vi "Agilent Scan EZ Temperature.vi"(0 "VISA Resource Name":refnum<visa-resource-name>, 2 "Control":enum16{"Initialize", "Read", "Experiment"}(ring), 5 "Channel Input":string, 11 "error in (no error)":errorcluster) -> (4 "VISA Resource Name Out":refnum<visa-resource-name>, 6 "read buffer":string, 8 "Output Array":dbl[](array[numeric]) format="%.2f", 15 "error out":errorcluster)   [LabVIEW 2012]
doc: "This VI lets you take simple temperature measurements. You can use various types of thermocouples, thermistors, or RTDs."
uses:
  Drivers/Agilent 34970/Agilent 34970.lvlib
panel:
  in  "Integration Time":u16(ring)=300 items=[".02 PLC"=10000, ".2 PLC"=1000, "1 PLC"=300, "2 PLC"=220, "10 PLC"=100, "20 PLC"=80, "100 PLC"=30, "200 PLC"=22]
  in  "AutoZero":bool
  out "Command":string
  out "Length":i32
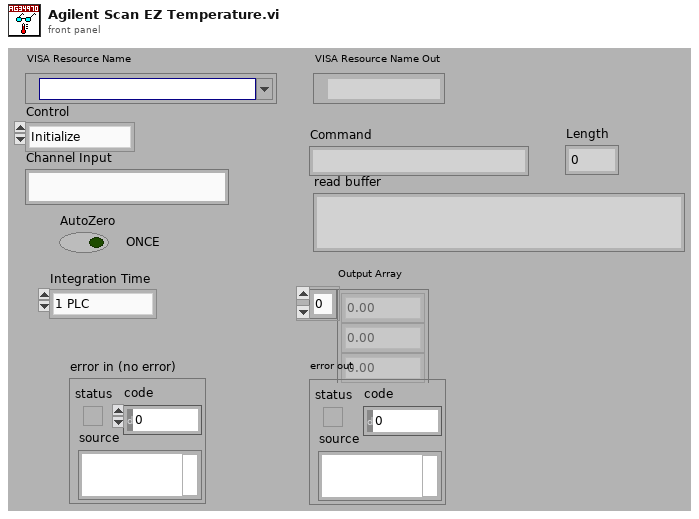
[diagram p1: front panel]
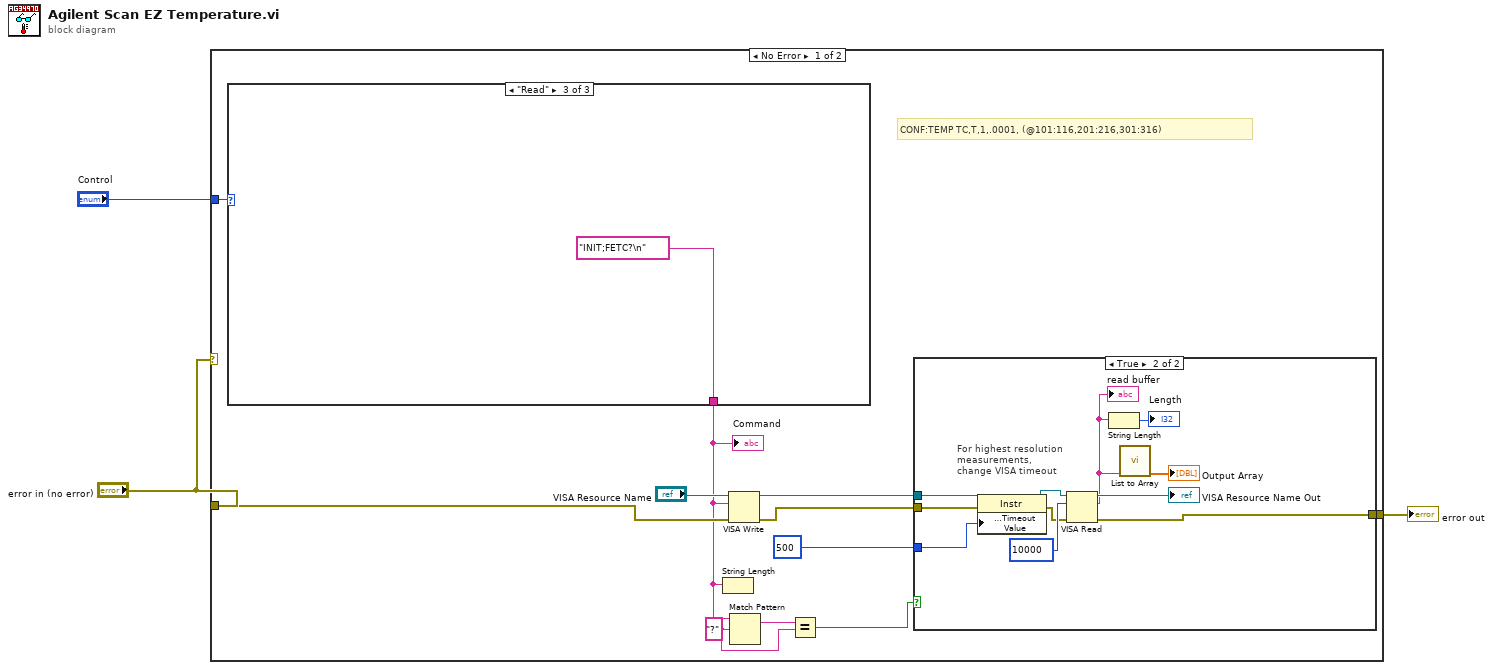
[diagram p0: block diagram]
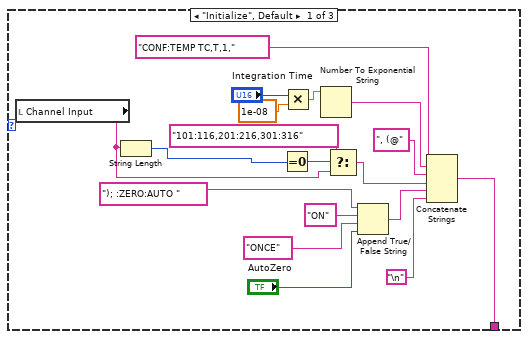
[diagram p3: hidden frame]
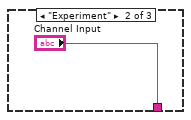
[diagram p4: hidden frame]
diagram:
  n1 = case shown="No Error" "error in (no error)" {
    tunnel: "error in (no error)" -> [w13 w47]
    tunnel: "Control" -> [w5 _]
    tunnel: [w4 w47] -> w1
    frame No Error {
      w7 = "?" ("regular expression")
      # "CONF:TEMP TC,T,1,.0001, (@101:116,201:216,301:316)"
      n2 = case shown="\"Read\"" w5 {
        tunnel: [w36 "Channel Input" "INIT;FETC?\n" ("0")] -> w9
        frame "Initialize", Default {
          n3 = local read "Channel Input"() -> (w29:string)
          n4 = String Length(string=w29) -> (length=w32:i32)
          n5 = Equal To 0?(x=w32) -> (x = 0?=w31:bool)
          n6 = Multiply(x="Integration Time", y=1e-08) -> (x*y=w39:dbl)
          n7 = Number To Exponential String(number=w39) -> (E-format string=w38:string)  [unwired: 3 in]
          n8 = Select(t="101:116,201:216,301:316" ("0"), s=w31, f=w29) -> (s? t:f=w28:string)
          n9 = Append True/False String(1:"AutoZero", 2:"ONCE" ("false string"), 3:"ON" ("true string"), 4:"); :ZERO:AUTO " ("0")) -> (0:w34:string)
          n10 = Concatenate Strings("CONF:TEMP TC,T,1," ("0"), w38, ", (@" ("0"), w28, w34, "\n") -> (w36:string)
        }
        frame "Experiment" {
        }
        frame "Read" {
        }
      }
      "Command" <- w9
      n11 = String Length(string=w9) -> ()  [unwired: 1 out]
      n12 = VISA Write(VISA resource name="VISA Resource Name", write buffer=w9, error in (no error)=w13) -> (VISA resource name out=w11:refnum<visa-resource-name>, error out=w10:errorcluster)  [unwired: 1 out]
      n13 = Match Pattern(string=w9, regular expression=w7) -> (match substring=w8:string)  [unwired: 1 in, 3 out]
      n14 = Equal?(x=w8, y=w7) -> (x = y?=w6:bool)
      n15 = case shown="True" w6 {
        tunnel: u32 500 ("Tmo Value") -> [_ w23]
        tunnel: w11 -> [_ w22]
        tunnel: w10 -> [w15 w21]
        tunnel: [w15 w16] -> w4
        frame False {
        }
        frame True {
          # "For highest resolution\nmeasurements, \nchange VISA timeout"
          n16 = property class="Instr"(reference=w22, error in=w21, "General Settings:Timeout Value"=w23) -> (reference out=w20:refnum<visa-resource-name>, error out=w19:errorcluster)
          n17 = VISA Read(VISA resource name=w20, byte count=u32 10000 ("byte count (0)"), error in (no error)=w19) -> (VISA resource name out=→"VISA Resource Name Out":refnum<visa-resource-name>, read buffer=w18:string, error out=w16:errorcluster)  [unwired: 1 out]
          "read buffer" <- w18
          n18 = String Length(string=w18) -> (length=→"Length":i32)
          n19 = call "List to Array.vi"("List (empty)"=w18) -> ("Output Number Array"=→"Output Array":dbl[])  [unwired: 9 in, 1 out]
        }
      }
    }
    frame Error {
    }
  }
  "error out" <- w1
